vi "Auto_Routine_Deposit.vi"(8 "error in (no error)":errorcluster, 9 "Distance From Grid":dbl, 10 "Game Piece":enum16{"Cube", "Cone"}(ring), 11 "Position":enum16{"Upper", "Lower", "Middle"}(ring)) -> (0 "error out":errorcluster)   [LabVIEW 2020]
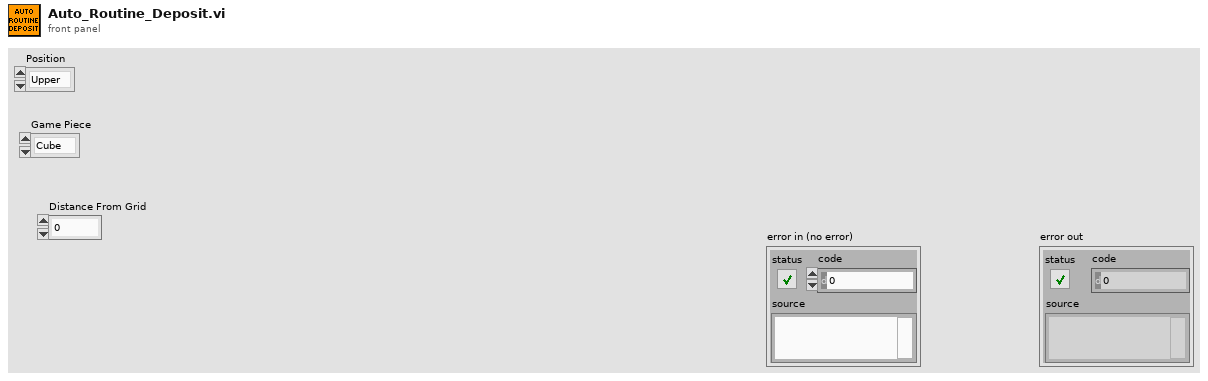
[diagram p1: front panel]
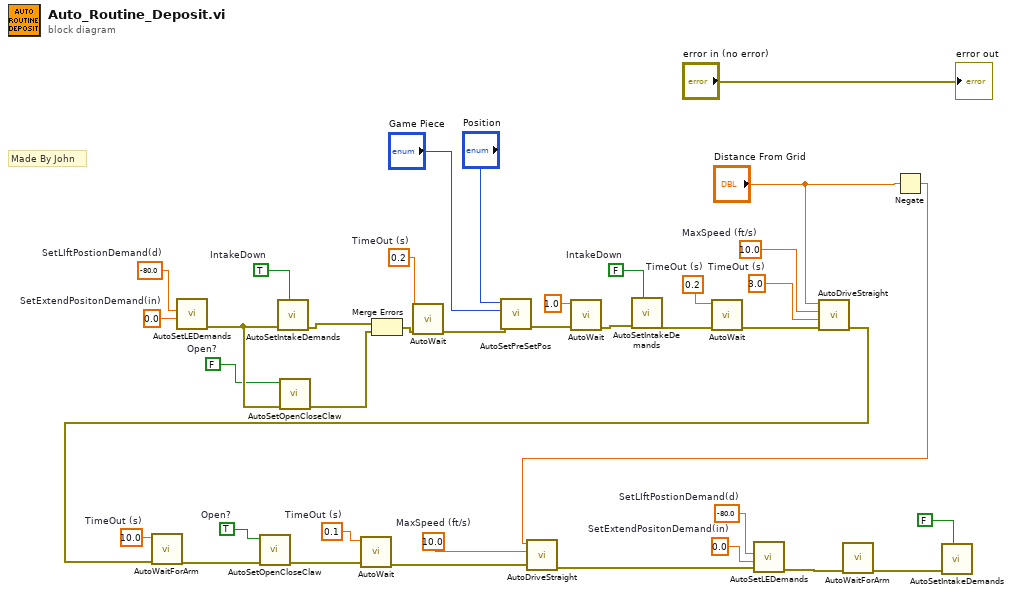
[diagram p0: block diagram]
diagram:
  w11 = -80.0  # SetLIftPostionDemand(d)
  w10 = 0.0  # SetExtendPositonDemand(in)
  w35 = 10.0  # MaxSpeed (ft/s)
  w31 = 3.0  # TimeOut (s)
  w30 = 10.0  # MaxSpeed (ft/s)
  w28 = 0.1  # TimeOut (s)
  w26 = TRUE  # Open?
  w24 = 0.2  # TimeOut (s)
  w23 = 10.0  # TimeOut (s)
  w18 = FALSE  # IntakeDown
  w16 = 0.2  # TimeOut (s)
  w15 = -80.0  # SetLIftPostionDemand(d)
  w14 = 0.0  # SetExtendPositonDemand(in)
  w13 = FALSE  # Open?
  w12 = TRUE  # IntakeDown
  # "Made By John"
  n1 = call "AutoSetLEDemands.vi"("SetExtendPositonDemand(in)"=w14, "SetLIftPostionDemand(d)"=w15) -> ("error out"=w20:errorcluster)  [unwired: 9 in]
  n2 = call "AutoSetIntakeDemands.vi"("IntakeDown"=w12, "error in (no error)"=w20) -> ("error out"=w32:errorcluster)  [unwired: 9 in]
  n3 = call "AutoSetOpenCloseClaw.vi"("error in (no error)"=w20, "Open?"=w13) -> ("error out"=w33:errorcluster)  [unwired: 9 in]
  n4 = Merge Errors(w32, w33) -> (w34:errorcluster)
  n5 = call "AutoWait.vi"("error in (no error)"=w34, "TimeOut (s)"=w16) -> ("error out"=w17:errorcluster)  [unwired: 9 in]
  n6 = call "AutoSetPreSetPos.vi"("error in (no error)"=w17, "Game Piece"="Game Piece", "Position"="Position") -> ("error out"=w36:errorcluster)  [unwired: 8 in]
  n7 = call "AutoWait.vi"("error in (no error)"=w36, "TimeOut (s)"=1.0) -> ("error out"=w37:errorcluster)  [unwired: 9 in]
  n8 = call "AutoSetIntakeDemands.vi"("IntakeDown"=w18, "error in (no error)"=w37) -> ("error out"=w19:errorcluster)  [unwired: 9 in]
  n9 = call "AutoWait.vi"("error in (no error)"=w19, "TimeOut (s)"=w24) -> ("error out"=w21:errorcluster)  [unwired: 9 in]
  n10 = call "AutoDriveStraight.vi"("error in (no error)"=w21, "TimeOut (s)"=w31, "MaxSpeed (ft/s)"=w30, "Dist (ft)"="Distance From Grid") -> ("error out"=w22:errorcluster)  [unwired: 7 in]
  n11 = call "AutoWaitForArm.vi"("error in (no error)"=w22, "TimeOut (s)"=w23) -> ("error out"=w25:errorcluster)  [unwired: 9 in]
  n12 = call "AutoSetOpenCloseClaw.vi"("error in (no error)"=w25, "Open?"=w26) -> ("error out"=w27:errorcluster)  [unwired: 9 in]
  n13 = call "AutoWait.vi"("error in (no error)"=w27, "TimeOut (s)"=w28) -> ("error out"=w29:errorcluster)  [unwired: 9 in]
  n14 = Negate(x="Distance From Grid") -> (-x=w1:dbl)
  n15 = call "AutoDriveStraight.vi"("error in (no error)"=w29, "MaxSpeed (ft/s)"=w35, "Dist (ft)"=w1) -> ("error out"=w9:errorcluster)  [unwired: 8 in]
  n16 = call "AutoSetLEDemands.vi"("error in (no error)"=w9, "SetExtendPositonDemand(in)"=w10, "SetLIftPostionDemand(d)"=w11) -> ("error out"=w8:errorcluster)  [unwired: 8 in]
  n17 = call "AutoWaitForArm.vi"("error in (no error)"=w8) -> ("error out"=w7:errorcluster)  [unwired: 10 in]
  n18 = call "AutoSetIntakeDemands.vi"("IntakeDown"=FALSE, "error in (no error)"=w7) -> ()  [unwired: 9 in, 1 out]
  "error out" <- "error in (no error)"
